vi "Create Device.vi"(8 "error in (no error)":errorcluster, 10 "Description":string, 11 "Name":string) -> (0 "error out":errorcluster, 3 "Custom Device":refnum<k24>)   [LabVIEW 2010, in "RefMem PtByPt System Definition API.lvlib"]
doc: "Creates a new instance of the Read Reflective Memory Point by Point Custom Device. This custom device reads reflective memory addresses point by point instaed of by DMA (the built-in NI VeriStand behavior)."
uses:
  RefMem PtByPt System Definition API.lvlib
  NationalInstruments.VeriStand.SystemDefinitionAPI
  Custom Device/Controls/Global.vi
  Custom Device/RefMem PtByPt Custom Device.lvlib
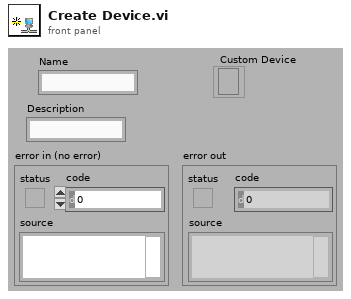
[diagram p1: front panel]
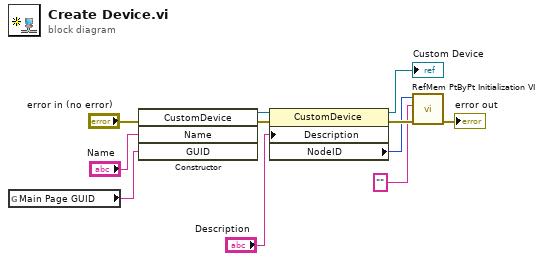
[diagram p0: block diagram]
diagram:
  n1 = global read "Global.vi" "Main Page GUID"() -> (w10:string)
  n2 = constructor class="CustomDevice"(error in="error in (no error)", "Name"="Name", "GUID"=w10) -> (reference out=w8:refnum<k24>, error out=w9:errorcluster)  [unwired: 2 in, 3 out]
  n3 = property class="CustomDevice"(reference=w8, error in=w9, "Description"="Description") -> (reference out=→"Custom Device":refnum<k24>, error out=w6:errorcluster, "NodeID"=w4:u64)
  n4 = call "RefMem PtByPt Initialization VI.vi"("error in (no error)"=w6, "Custom XML"="", "Device Item Ref in"=w4) -> ("error out"=→"error out":errorcluster)  [unwired: 7 in, 1 out]
